vi "Store Voltage Measurement.vi"(8 "error in":errorcluster, 10 "Value":dbl, 11 "Measurement":T1) -> (0 "error out":errorcluster)   [LabVIEW 2016, in "Hall Effect Library.lvlib"]
uses:
  Hall Effect Library.lvlib
  Controls/Measurement.ctl
  Global Variables/Hall Effect Data.vi
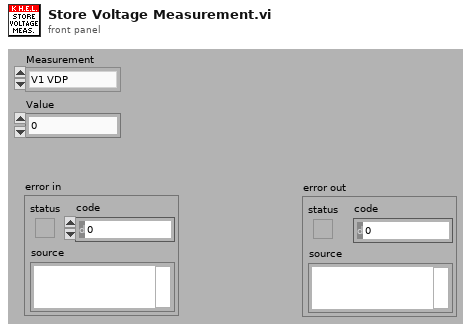
[diagram p1: front panel]
types:
  T1 = typedef "Hall Effect Library.lvlib/Measurement.ctl" = enum16{"V1 VDP", "V2 VDP", "V3 VDP", "V4 VDP", "V5 VDP", "V6 VDP", "V7 VDP", "V8 VDP", "V1 HE", "V2 HE", "V3 HE", "V4 HE", "V5 HE", "V6 HE", "V7 HE", "V8 HE", "V1 Res Bar", "V1 Hall Bar", "V1 Res 6-Cot", "V2 Res 6-Cot", "V3 Res 6-Cot", "V4 Res 6-Cot", "V1 Hall 6-Cot", "V2 Hall 6-Cot", "V3 Hall 6-Cot", "V4 Hall 6-Cot", "V5 Hall 6-Cot", "V6 Hall 6-Cot", "V7 Hall 6-Cot", "V8 Hall 6-Cot", "V1 Res 8-Cot", "V2 Res 8-Cot", "V3 Res 8-Cot", "V4 Res 8-Cot", "V1 Hall 8-Cot", "V2 Hall 8-Cot", "V3 Hall 8-Cot", "V4 Hall 8-Cot"}
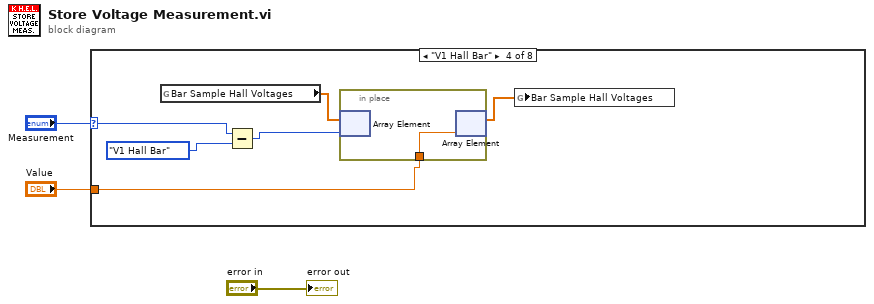
[diagram p0: block diagram]
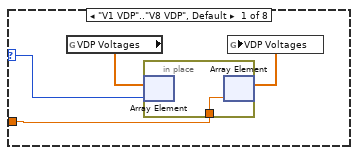
[diagram p2: hidden frame]
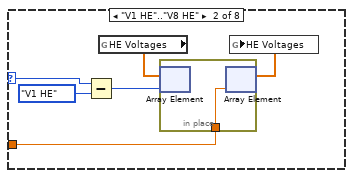
[diagram p3: hidden frame]
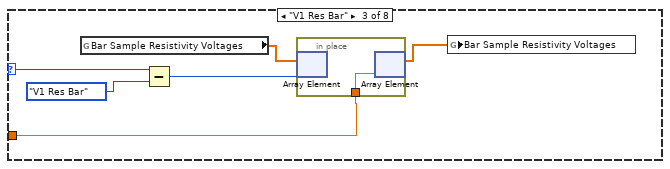
[diagram p4: hidden frame]
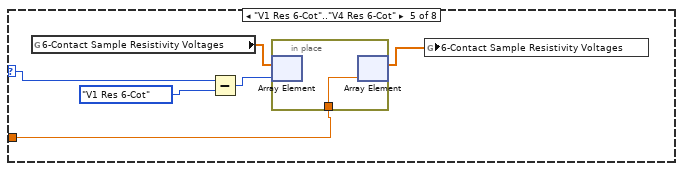
[diagram p5: hidden frame]
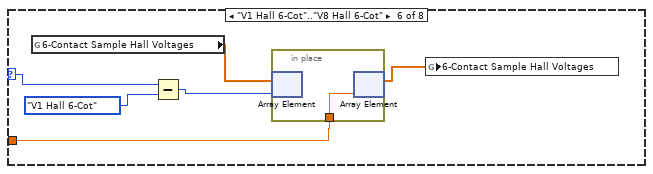
[diagram p6: hidden frame]
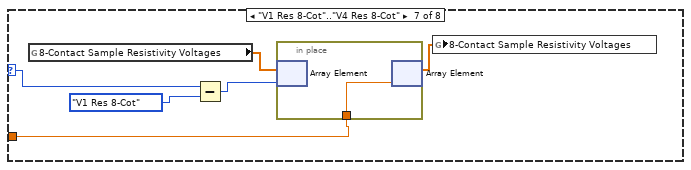
[diagram p7: hidden frame]
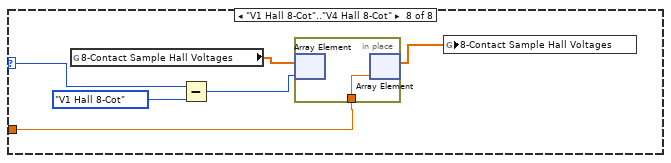
[diagram p8: hidden frame]
diagram:
  n1 = case shown="\"V1 Hall Bar\"" "Measurement" {
    selector: "Measurement" -> [w6 w12 w18 w26 w31 w38 w45 w52]
    tunnel: "Value" -> [w5 w9 w19 w27 w33 w40 w47 w54]
    frame "V1 VDP".."V8 VDP", Default {
      n2 = global read "Hall Effect Data.vi" "VDP Voltages"() -> (w7:dbl[])
      n3 = in-place {
        in-place-border: w5 -> [w8]
        n4 = in-place-array #1(w7, w6) -> ()  [unwired: 1 out]
        n5 = in-place-array #1(w8) -> (w4:dbl[])  [unwired: 1 out]
      }
      n6 = global write "Hall Effect Data.vi" "VDP Voltages"(w4) -> ()
    }
    frame "V1 HE".."V8 HE" {
      n7 = Subtract(x=w12, y=Measurement."V1 HE") -> (x-y=w10:u16)
      n8 = global read "Hall Effect Data.vi" "HE Voltages"() -> (w14:dbl[])
      n9 = in-place {
        in-place-border: w9 -> [w15]
        n10 = in-place-array #2(w14, w10) -> ()  [unwired: 1 out]
        n11 = in-place-array #2(w15) -> (w13:dbl[])  [unwired: 1 out]
      }
      n12 = global write "Hall Effect Data.vi" "HE Voltages"(w13) -> ()
    }
    frame "V1 Res Bar" {
      n13 = global read "Hall Effect Data.vi" "Bar Sample Resistivity Voltages"() -> (w21:dbl[])
      n14 = Subtract(x=w18, y=Measurement."V1 Res Bar") -> (x-y=w16:u16)
      n15 = in-place {
        in-place-border: w19 -> [w22]
        n16 = in-place-array #3(w21, w16) -> ()  [unwired: 1 out]
        n17 = in-place-array #3(w22) -> (w20:dbl[])  [unwired: 1 out]
      }
      n18 = global write "Hall Effect Data.vi" "Bar Sample Resistivity Voltages"(w20) -> ()
    }
    frame "V1 Hall Bar" {
      n19 = global read "Hall Effect Data.vi" "Bar Sample Hall Voltages"() -> (w28:dbl[])
      n20 = Subtract(x=w26, y=Measurement."V1 Hall Bar") -> (x-y=w25:u16)
      n21 = in-place {
        in-place-border: w27 -> [w29]
        n22 = in-place-array #4(w28, w25) -> ()  [unwired: 1 out]
        n23 = in-place-array #4(w29) -> (w24:dbl[])  [unwired: 1 out]
      }
      n24 = global write "Hall Effect Data.vi" "Bar Sample Hall Voltages"(w24) -> ()
    }
    frame "V1 Res 6-Cot".."V4 Res 6-Cot" {
      n25 = global read "Hall Effect Data.vi" "6-Contact Sample Resistivity Voltages"() -> (w35:dbl[])
      n26 = Subtract(x=w31, y=Measurement."V1 Res 6-Cot") -> (x-y=w30:u16)
      n27 = in-place {
        in-place-border: w33 -> [w36]
        n28 = in-place-array #5(w35, w30) -> ()  [unwired: 1 out]
        n29 = in-place-array #5(w36) -> (w34:dbl[])  [unwired: 1 out]
      }
      n30 = global write "Hall Effect Data.vi" "6-Contact Sample Resistivity Voltages"(w34) -> ()
    }
    frame "V1 Hall 6-Cot".."V8 Hall 6-Cot" {
      n31 = global read "Hall Effect Data.vi" "6-Contact Sample Hall Voltages"() -> (w41:dbl[])
      n32 = Subtract(x=w38, y=Measurement."V1 Hall 6-Cot") -> (x-y=w37:u16)
      n33 = in-place {
        in-place-border: w40 -> [w43]
        n34 = in-place-array #6(w41, w37) -> ()  [unwired: 1 out]
        n35 = in-place-array #6(w43) -> (w42:dbl[])  [unwired: 1 out]
      }
      n36 = global write "Hall Effect Data.vi" "6-Contact Sample Hall Voltages"(w42) -> ()
    }
    frame "V1 Res 8-Cot".."V4 Res 8-Cot" {
      n37 = global read "Hall Effect Data.vi" "8-Contact Sample Resistivity Voltages"() -> (w48:dbl[])
      n38 = Subtract(x=w45, y=Measurement."V1 Res 8-Cot") -> (x-y=w44:u16)
      n39 = in-place {
        in-place-border: w47 -> [w50]
        n40 = in-place-array #7(w48, w44) -> ()  [unwired: 1 out]
        n41 = in-place-array #7(w50) -> (w49:dbl[])  [unwired: 1 out]
      }
      n42 = global write "Hall Effect Data.vi" "8-Contact Sample Resistivity Voltages"(w49) -> ()
    }
    frame "V1 Hall 8-Cot".."V4 Hall 8-Cot" {
      n43 = global read "Hall Effect Data.vi" "8-Contact Sample Hall Voltages"() -> (w56:dbl[])
      n44 = Subtract(x=w52, y=Measurement."V1 Hall 8-Cot") -> (x-y=w51:u16)
      n45 = in-place {
        in-place-border: w54 -> [w57]
        n46 = in-place-array #8(w56, w51) -> ()  [unwired: 1 out]
        n47 = in-place-array #8(w57) -> (w55:dbl[])  [unwired: 1 out]
      }
      n48 = global write "Hall Effect Data.vi" "8-Contact Sample Hall Voltages"(w55) -> ()
    }
  }
  "error out" <- "error in"
